vi "NFILE3.vi"() -> ()   [LabVIEW 2019]
uses:
  Control 3.ctl
  Control 1.ctl
  <vilib>/Analysis/5stat.llb/RMS (DBL).vi
  <vilib>/Analysis/NI_AALPro.lvlib
panel:
  in  "stop":bool
  out "Urms":dbl format="%0.2f"
  out "Triggered signal":cluster{dbl[], "Vstupní pole":dbl[]}(graph)
  out "Staticky signal v casovem okne":dbl[](graph)
  out "XY Graph":cluster{dbl[], "Vstupní pole":dbl[]}(graph)
  in  "Úroven filtrace":i32
  out "SamInWin":i32
  in  "Frekvence":dbl=10.0 format="%0.2p"
  in  "Amplituda":dbl=1.0 format="%0.2p"
  in  "Amplituda sumu":T1
  in  "Offset":dbl format="%0.2p"
  in  "Sirka okna (ms)":i32(listbox)
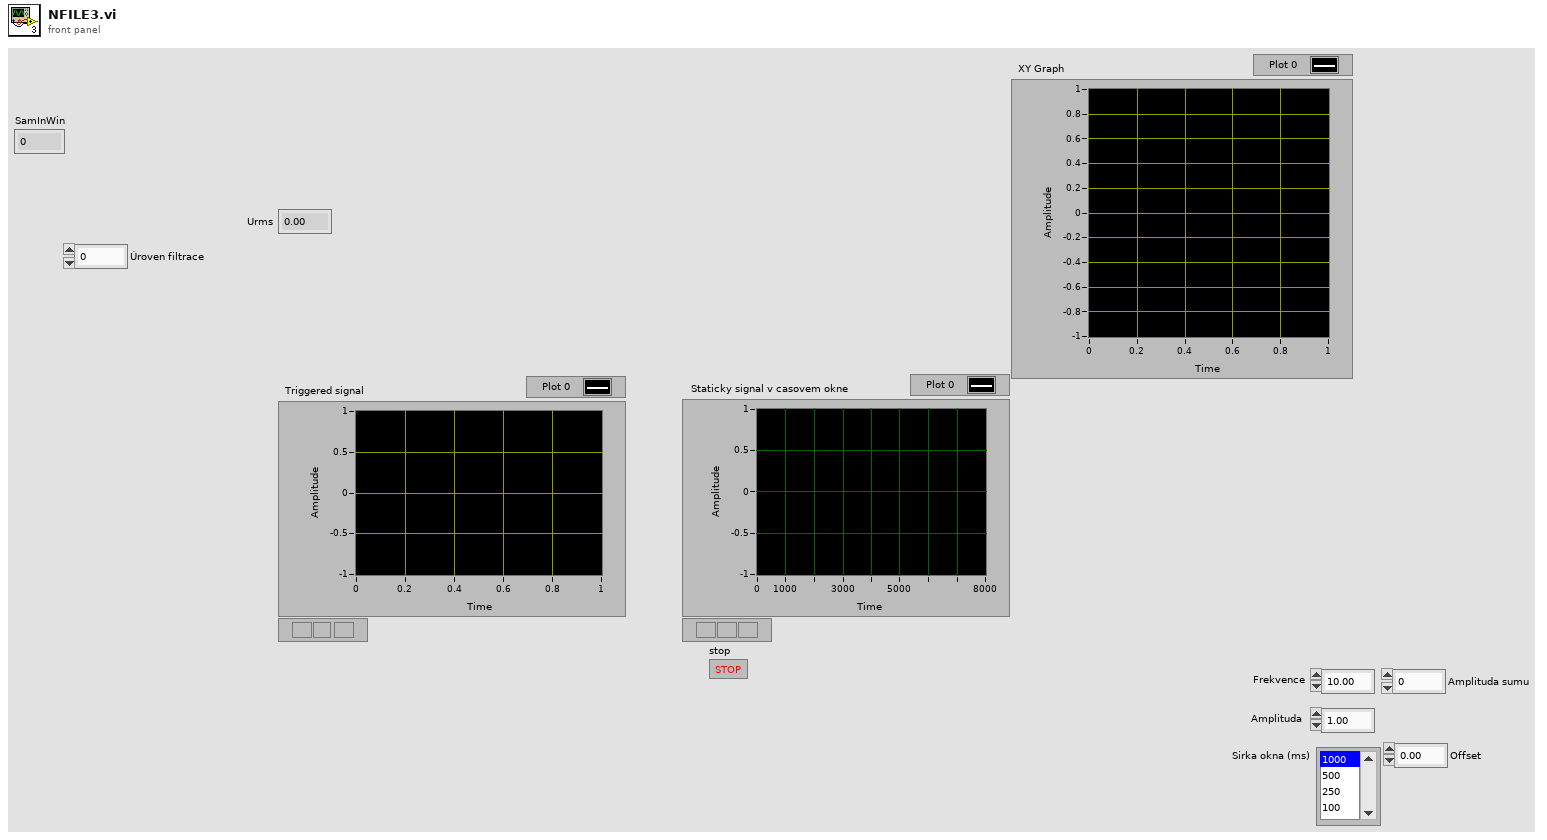
[diagram p1: front panel]
types:
  T1 = typedef "Control 3.ctl" = dbl
  T2 = typedef "Control 1.ctl" = dbl
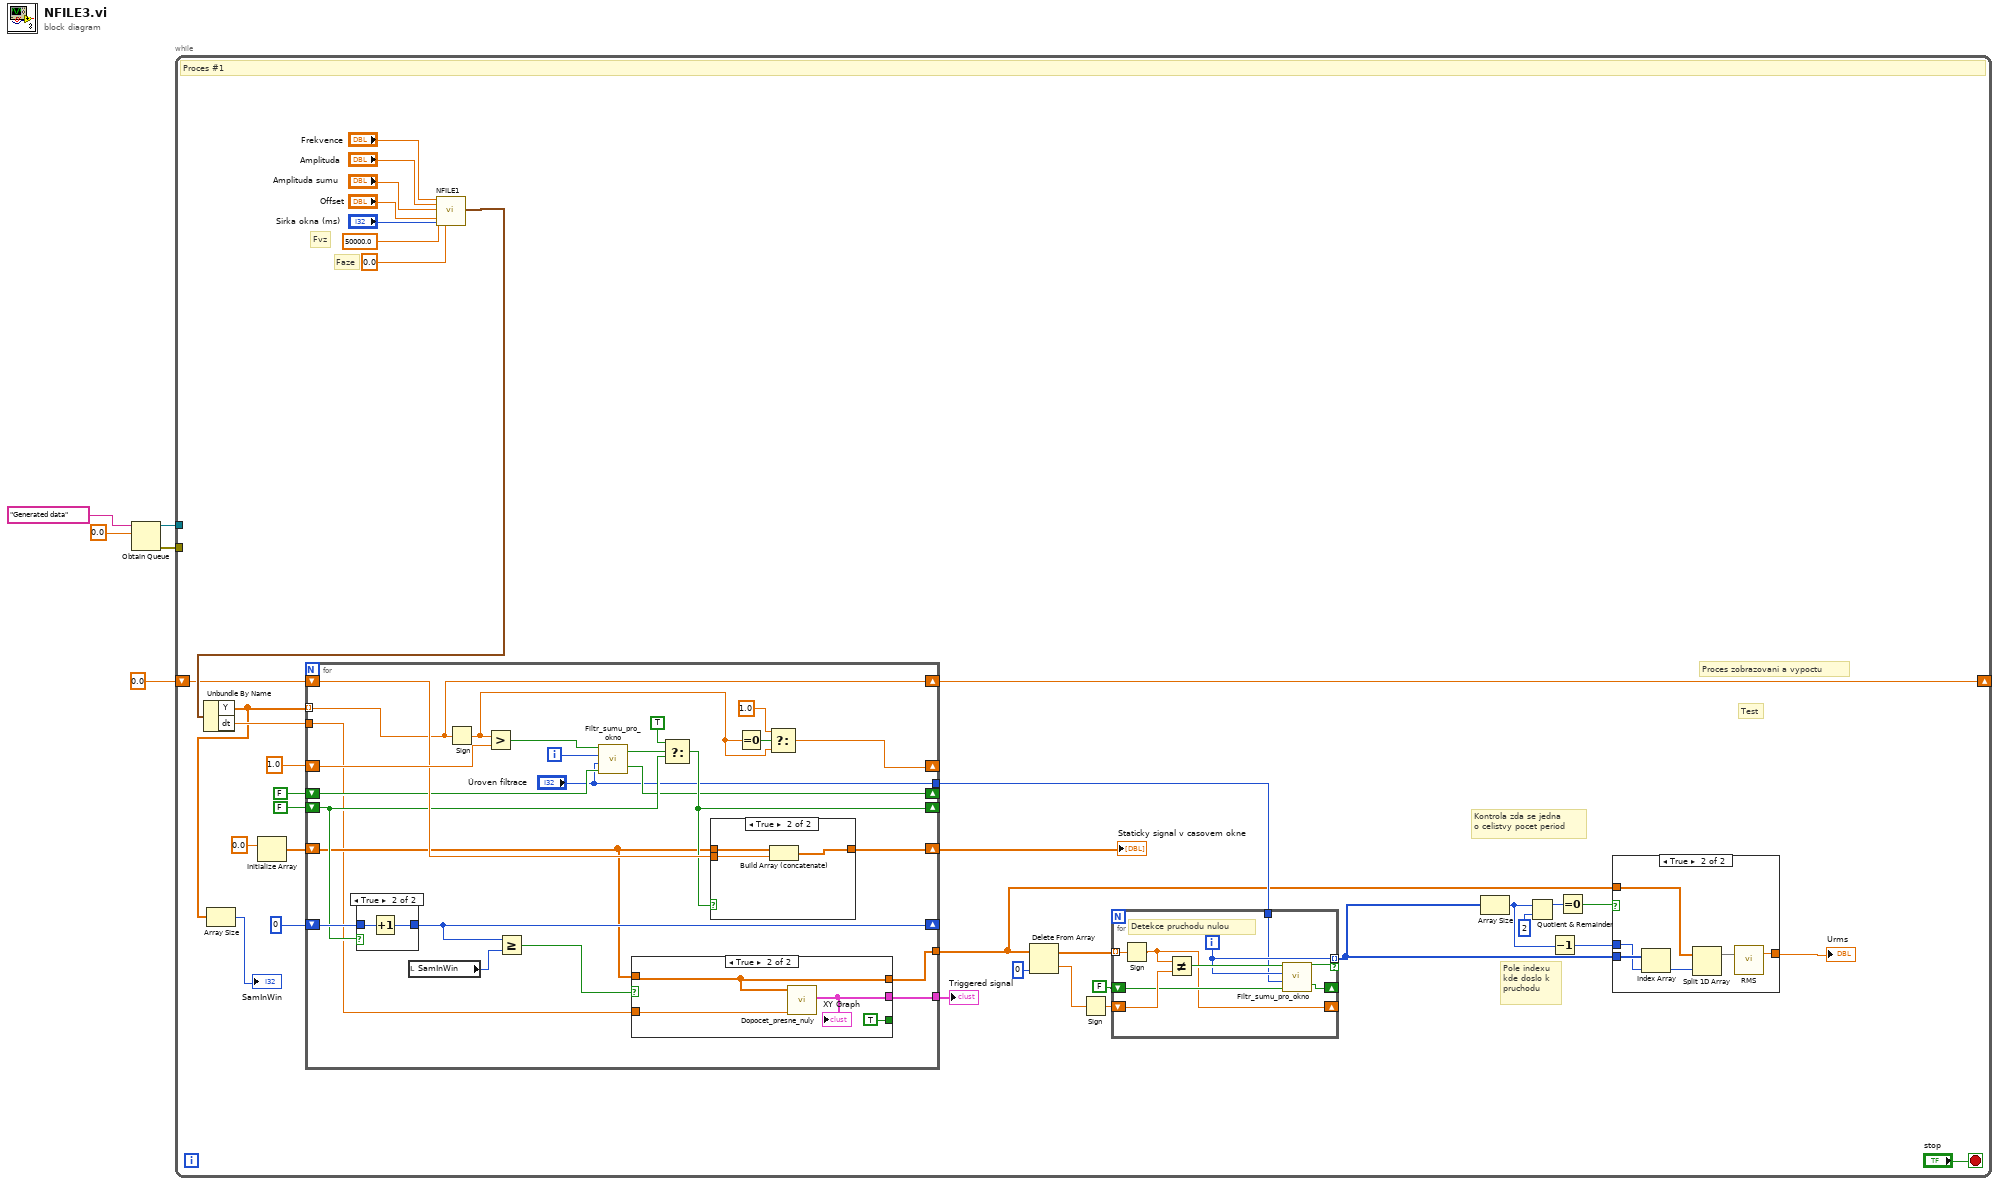
[diagram p0: block diagram]
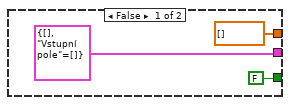
[diagram p2: hidden frame]
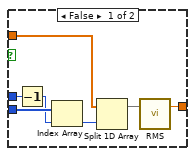
[diagram p5: hidden frame]
diagram:
  n1 = Obtain Queue(name (unnamed)="Generated data", element data type=0.0) -> (queue out=w3:refnum<queue>, error out=w2:errorcluster)  [unwired: 3 in, 1 out]
  n2 = while {
    tunnel: w3 -> [_]
    tunnel: w2 -> [_]
    shift-right: [w10] -> _
    shift-left: 0.0 ("element") -> [w11]
    stop <- "stop" stop-if-true
    # "Proces zobrazovani a vypoctu"
    # "Kontrola zda se jedna\no celistvy pocet period"
    # "Pole indexu\nkde doslo k\npruchodu"
    # "Test"
    # "Fvz"
    # "Faze"
    # "Proces #1"
    n3 = Initialize Array(0.0 ("element")) -> (w31:dbl[])  [unwired: 1 in]
    n4 = call "NFILE1.vi"("Frekvence"="Frekvence", "Amplituda"="Amplituda", "Amplituda sumu"="Amplituda sumu", "Fáze"=0.0, "Offset"="Offset", "Sirka okna (ms)"="Sirka okna (ms)", "Fvz"=T2 50000.0) -> ("Waveform Graph"=w34:waveform(dbl))  [unwired: 12 in]
    n5 = Unbundle By Name(w34) -> ("Y"=w8:dbl[], "dt"=w9:dbl)
    n6 = Array Size(array=w8) -> (size(s)=→"SamInWin":i32)
    n7 = for {
      shift-right: [w48] -> _
      shift-left: 1.0 -> [w66]
      shift-right: [w62] -> _
      shift-left: 0 -> [w64]
      shift-right: [w47] -> w27
      shift-left: w31 -> [w44]
      tunnel: [w61] -> w30
      shift-right: [w58] -> _
      shift-left: FALSE -> [w59]
      shift-right: [w43] -> w10
      shift-left: w11 -> [w60]
      shift-right: [w54] -> _
      shift-left: FALSE -> [w55]
      tunnel: [w46] -> w26
      tunnel: ["Úroven filtrace"] -> w15
      tunnel: w8 -> [w43] mode=indexing
      tunnel: w9 -> [w42]
      i -> [w56]
      n8 = case shown="True" w59 {
        tunnel: w64 -> [w74 w76]
        tunnel: [w74 w75] -> w62
        frame False {
        }
        frame True {
          n9 = Increment(x=w76) -> (x+1=w75:i32)
        }
      }
      n10 = local read "SamInWin"() -> (w63:i32)
      n11 = Sign(1:w43) -> (0:w49:dbl)
      n12 = Greater?(x=w49, y=w66) -> (0:w57:bool)
      n13 = Greater Or Equal?(x=w62, y=w63) -> (x >= y?=w52:bool)
      n14 = call "Filtr_sumu_pro_okno.vi"("ShiftIn"=w55, "Citlivost 2"="Úroven filtrace", "i"=w56, "trig_in"=w57) -> ("ShiftOut"=w54:bool, "trig_out"=w53:bool)
      n15 = case shown="True" w52 {
        tunnel: [FALSE TRUE] -> _
        tunnel: w44 -> [_ w71]
        tunnel: [cluster{dbl[], "Vstupní pole":dbl[]} {[], "Vstupní pole"=[]} ("XY Graph 2") w72] -> w61
        tunnel: [dbl[] [] w71] -> w46
        tunnel: w42 -> [_ w70]
        frame False {
        }
        frame True {
          n16 = call "Dopocet_presne_nuly.vi"("dt"=w70, "Vstupní pole"=w71) -> ("XY Graph"=w72:cluster{dbl[], "Vstupní pole":dbl[]})  [unwired: 9 in]
          "XY Graph" <- w72
        }
      }
      n17 = Select(t=TRUE, s=w53, f=w59) -> (s? t:f=w58:bool)
      n18 = case shown="True" w58 {
        tunnel: w44 -> [w77 w80]
        tunnel: w60 -> [_ w79]
        tunnel: [w77 w78] -> w47
        frame False {
        }
        frame True {
          n19 = Build Array (concatenate)(w80, w79) -> (w78:dbl[])
        }
      }
      n20 = Equal To 0?(x=w49) -> (x = 0?=w51:bool)
      n21 = Select(t=1.0, s=w51, f=w49) -> (s? t:f=w48:dbl)
    }
    "Staticky signal v casovem okne" <- w27
    "Triggered signal" <- w30
    n22 = Delete From Array(array=w26, index=0) -> (deleted portion=w20:dbl, array with subset deleted=w13:dbl[])  [unwired: 1 in]
    n23 = Sign(1:w20) -> (0:w19:dbl)
    n24 = for {
      tunnel: w13 -> [w96] mode=indexing
      shift-right: [w95] -> _
      shift-left: w19 -> [w102]
      tunnel: [w99] -> w22 mode=indexing if=w100
      shift-right: [w97] -> _
      shift-left: FALSE -> [w98]
      tunnel: w15 -> [w94]
      i -> [w99]
      # "Detekce pruchodu nulou"
      n25 = Sign(1:w96) -> (0:w95:dbl)
      n26 = Not Equal?(x=w95, y=w102) -> (x != y?=w101:bool)
      n27 = call "Filtr_sumu_pro_okno.vi"("ShiftIn"=w98, "Citlivost 2"=w94, "i"=w99, "trig_in"=w101) -> ("ShiftOut"=w97:bool, "trig_out"=w100:bool)
    }
    n28 = Array Size(array=w22) -> (size(s)=w18:i32)
    n29 = Quotient & Remainder(x=w18, y=2) -> (x-y*floor(x/y)=w23:i32)  [unwired: 1 out]
    n30 = Decrement(x=w18) -> (x-1=w17:i32)
    n31 = Equal To 0?(x=w23) -> (x = 0?=w12:bool)
    n32 = case shown="True" w12 {
      tunnel: w17 -> [w85 w90]
      tunnel: w22 -> [w87 w93]
      tunnel: w13 -> [w81 w91]
      tunnel: [w82 w88] -> w14
      frame False {
        n33 = Decrement(x=w85) -> (x-1=w84:i32)
        n34 = Index Array(array=w87, index=w84) -> (element=w86:i32)
        n35 = Split 1D Array(array=w81, index=w86) -> (first subarray=w83:dbl[])  [unwired: 1 out]
        n36 = call-poly <vilib>:"RMS.vi"("X"=w83) -> ("rms value"=w82:dbl)  [unwired: 1 out]
      }
      frame True {
        n37 = Index Array(array=w93, index=w90) -> (element=w92:i32)
        n38 = Split 1D Array(array=w91, index=w92) -> (first subarray=w89:dbl[])  [unwired: 1 out]
        n39 = call-poly <vilib>:"RMS.vi"("X"=w89) -> ("rms value"=w88:dbl)  [unwired: 1 out]
      }
    }
    "Urms" <- w14
  }
